vi "LIN EX Init.vi"(7 "MasterMode":u8, 9 "BaudRate":u32, 10 "LINIndex":u8, 11 "DevHandle":i32) -> (3 "function return":i32)   [LabVIEW 2010, in "usb2lin_ex.lvlib"]
doc: "int WINAPI LIN_EX_Init(int DevHandle,unsigned char LINIndex,unsigned int BaudRate,unsigned char MasterMode);"
uses:
  usb2lin_ex.lvlib
  USB2XXX.dll
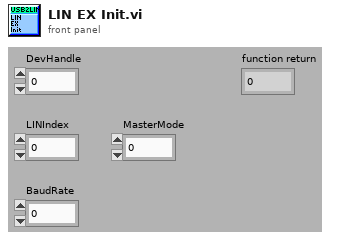
[diagram p1: front panel]
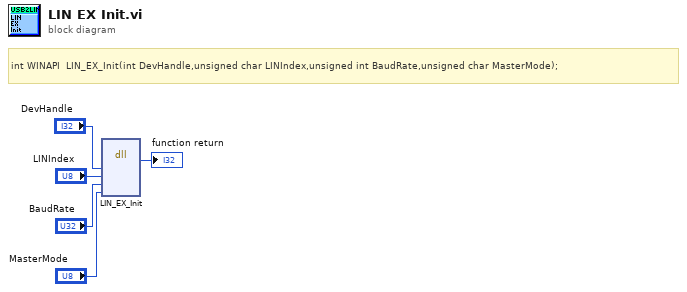
[diagram p0: block diagram]
diagram:
  # "int WINAPI  LIN_EX_Init(int DevHandle,unsigned char LINIndex,unsigned int BaudRate,unsigned char MasterMode);"
  n1 = dll-call lib="E:/OtherWork/STM32/USB2XXX_Example/sdk/api/Labview/USB2XXX.*" fn="LIN_EX_Init"("DevHandle"="DevHandle", "LINIndex"="LINIndex", "BaudRate"="BaudRate", "MasterMode"="MasterMode") -> (→"function return":i32)  [unwired: 7 in, 2 out]
